vi "热敏电阻多通道数据采集 - 副本.vi"() -> ()   [LabVIEW 2015]
uses:
  <vilib>/Utility/miscctls.llb/LVRowAndColumnTypeDef.ctl
  <vilib>/addons/_office/_exclsub.llb/font.ctl
  <vilib>/addons/_office/excel.llb/Excel Easy Table (str).vi
  <vilib>/Utility/NIReport.llb/NI_report.lvclass
  Keithley 27XX/Keithley 27XX.lvlib
  <vilib>/addons/_office/NI_ReportGenerationToolkit.lvlib
panel:
  out "数据显示 3":string[][](table)
  in  "Quit":bool
  out "队列输出":refnum<queue>
  out "采集使能":bool
  out "数据显示":string[][](table)
  in  "tab":enum32{"总线检查", "配置", "数据显示"}(tab)
  in  "Keithley2750":refnum<visa-resource-name>="COM3"
  in  "总线检查":bool
  in  "温度设置":bool
  in  "编号设置":bool
  in  "清空表格":bool
  in  "暂停":bool
  in  "采集温度":bool
  in  "目标温度":string(combo)
  in  "实测温度":string
  in  "生成报告":bool
  out "通道号":i32
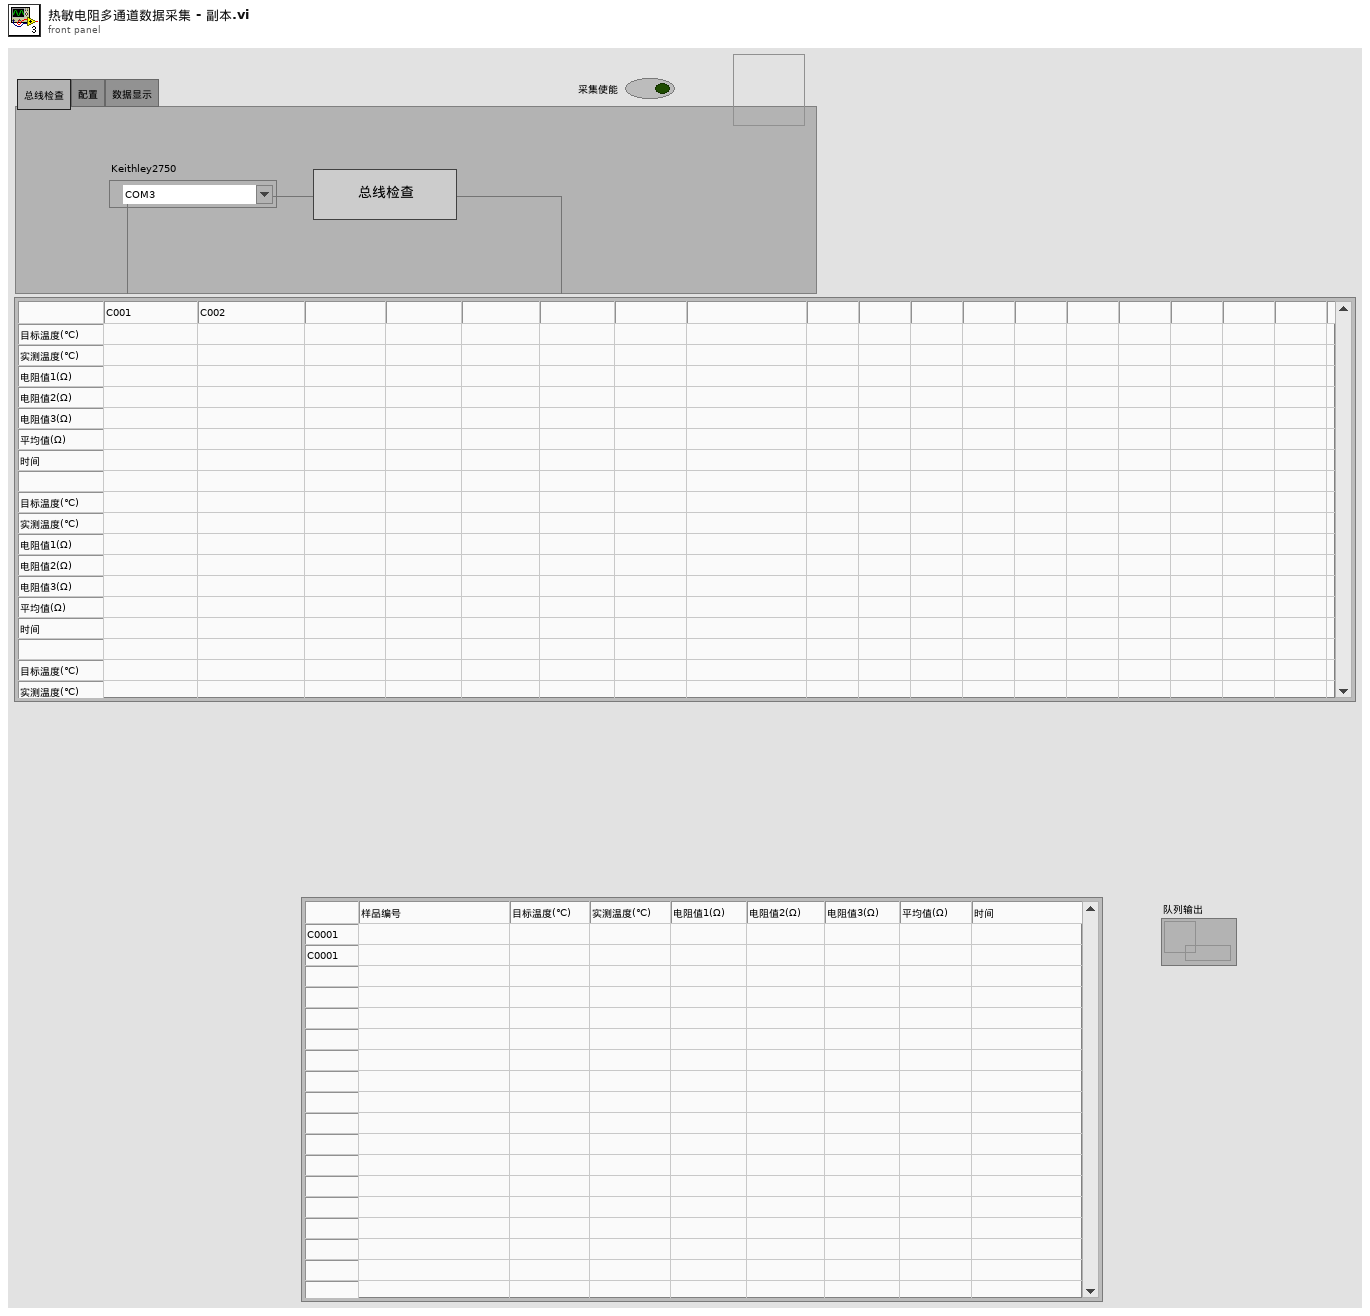
[diagram p1: front panel]
types:
  T1 = cluster{"Baud Rate (9600)":u32, "Flow Control (1: XON/XOFF)":u16, "Termination Char (0:CR)":u16}
  T2 = typedef "LVRowAndColumnTypeDef.ctl" = cluster{"Row":i32, "Column":i32}
  T3 = enum8{"Enabled", "Disabled", "Disabled and Grayed Out"}
  T4 = enum16{"maximized", "minimized", "normal", "no change"}
  T5 = enum16{"Standard Report", "HTML", "Word", "Excel"}
  T6 = typedef "NI_ReportGenerationToolkit.lvlib/font.ctl" = cluster{"font name":string, "font size":dbl, "bold":u16, "italic":u16, "underline":u16, "strike through":u16, "font color":u32}
  T7 = typedef "LVPoint32TypeDef.ctl" = cluster{"Horizontal":i32, "Vertical":i32}
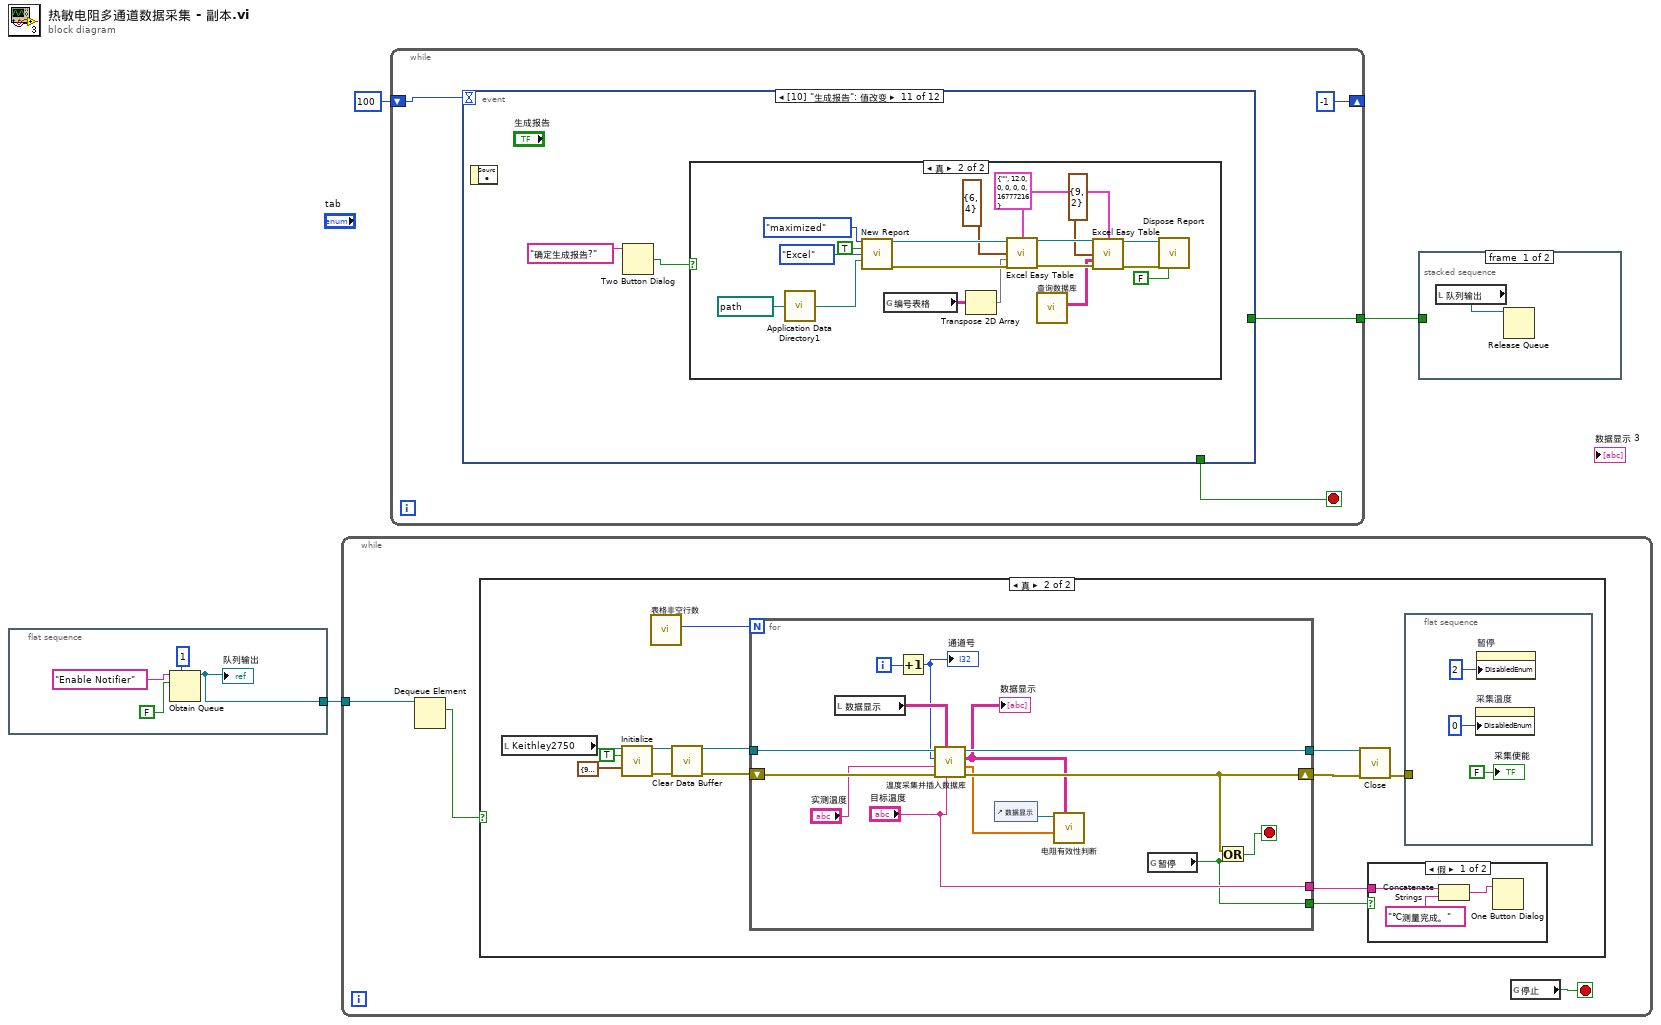
[diagram p0: block diagram]
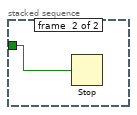
[diagram p2: hidden frame]
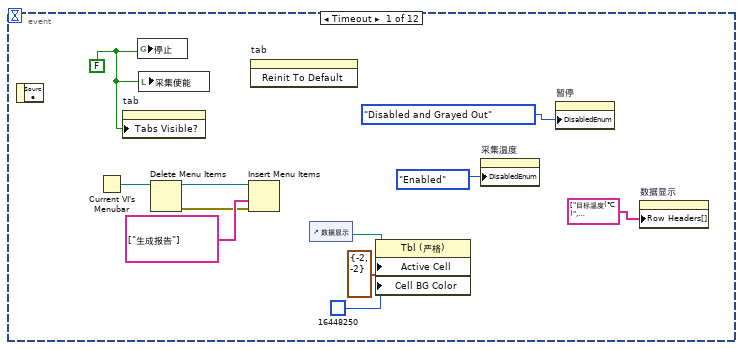
[diagram p5: hidden frame]
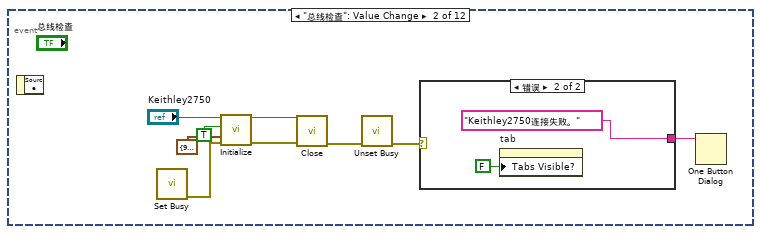
[diagram p6: hidden frame]
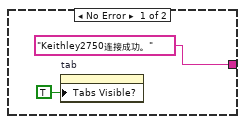
[diagram p7: hidden frame]
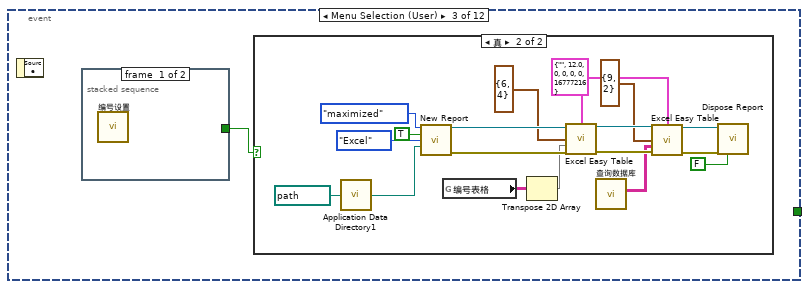
[diagram p8: hidden frame]
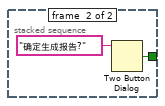
[diagram p9: hidden frame]
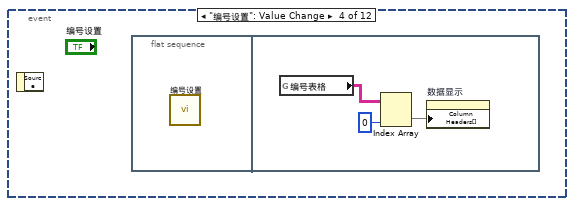
[diagram p11: hidden frame]
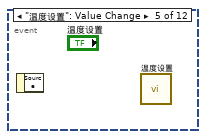
[diagram p12: hidden frame]
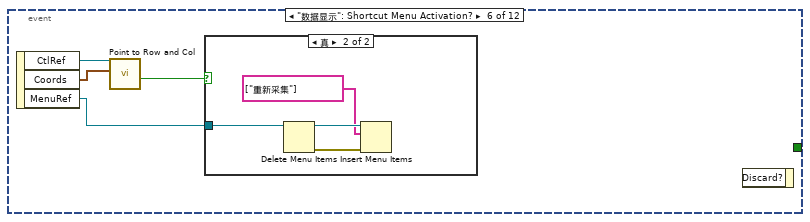
[diagram p13: hidden frame]
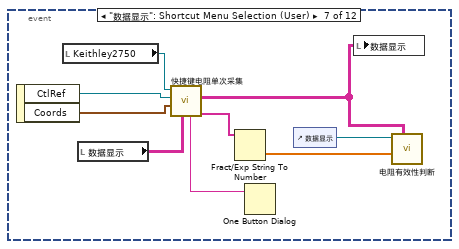
[diagram p15: hidden frame]
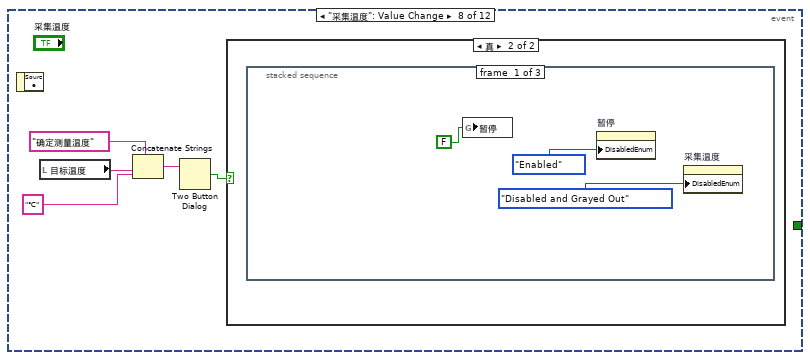
[diagram p16: hidden frame]
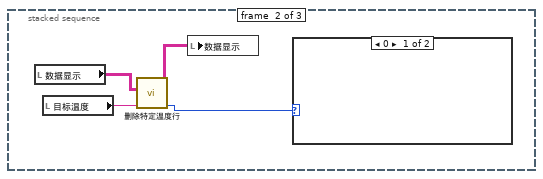
[diagram p18: hidden frame]
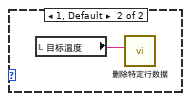
[diagram p19: hidden frame]
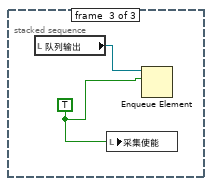
[diagram p20: hidden frame]
diagram:
  n1 = flat-sequence {
    tunnel: [w4] -> w1
    frame #0 {
      n2 = Obtain Queue(max queue size (-1, unlimited)=1 ("队列最大值（-1，无限）"), name (unnamed)="Enable Notifier", element data type=FALSE ("stop confirmed")) -> (queue out=w4:refnum<queue>)  [unwired: 2 in, 2 out]
      "队列输出" <- w4
    }
  }
  n3 = while {
    tunnel: w1 -> [w9]
    stop <- w10 stop-if-true
    n4 = Dequeue Element(queue=w9) -> (element=w8:bool)  [unwired: 2 in, 3 out]
    n5 = case shown="真" w8 {
      frame False {
      }
      frame True {
        n6 = local read "Keithley2750"() -> (w23:refnum<visa-resource-name>)
        n7 = call "Initialize.vi"("VISA resource name"=w23, "ID Query? (T: Yes)"=TRUE, "Serial Configuration"=T1 {"Baud Rate (9600)"=9600, "Flow Control (1: XON/XOFF)"=1, "Termination Char (0:CR)"=0}) -> ("VISA resource name out"=w21:refnum<visa-resource-name>, "error out"=w20:errorcluster)  [unwired: 11 in]
        n8 = call "表格非空行数.vi"() -> ("行数"=w12:i32)  [unwired: 11 in]
        n9 = call "Clear Data Buffer.vi"("VISA resource name"=w21, "error in (no error)"=w20) -> ("VISA resource name out"=w18:refnum<visa-resource-name>, "error out"=w19:errorcluster)  [unwired: 12 in]
        n10 = for {
          N: w12 -> [_]
          shift-right: [w40] -> w17
          shift-left: w19 -> [w43]
          tunnel: ["目标温度"] -> w13
          tunnel: w18 -> [w42]
          tunnel: [w41] -> w16
          tunnel: [w31] -> w11
          i -> [w32]
          stop <- w39 stop-if-true
          n11 = local read "数据显示"() -> (w34:string[][])
          n12 = Increment(x=w32) -> (x+1=w30:i32)
          "通道号" <- w30
          n13 = call "温度采集并插入数据库.vi"("目标温度"="目标温度", "数据显示1"=w34, "错误输入（无错误）"=w43, "实测温度"="实测温度", "通道号"=w30, "VISA引用句柄输入"=w42) -> ("错误输出"=w40:errorcluster, "温度值s"=w36:dbl[], "数据显示2"=w35:string[][], "VISA引用句柄输出"=w41:refnum<visa-resource-name>)  [unwired: 2 in]
          "数据显示" <- w35
          n14 = control-ref of="数据显示"() -> (w37:refnum<vi>)
          n15 = call "电阻有效性判断.vi"("数据显示"=w35, "温度值s"=w36, "Table输入"=w37) -> ()  [unwired: 9 in]
          n16 = global read "全局.vi" "暂停"() -> (w31:bool)
          n17 = Or(x=w40, y=w31) -> (x .or. y?=w39:bool)
        }
        n18 = call "Close.vi"("VISA resource name"=w16, "error in (no error)"=w17) -> ("error out"=w15:errorcluster)  [unwired: 13 in]
        n19 = case shown="假" w11 {
          tunnel: w13 -> [w26 _]
          frame False {
            n20 = Concatenate Strings(w26, "℃测量完成。") -> (w24:string)
            n21 = One Button Dialog(message=w24) -> ()  [unwired: 1 in, 1 out]
          }
          frame True {
          }
        }
        n22 = flat-sequence {
          tunnel: w15 -> [_]
          frame #0 {
            n23 = property on="采集温度" class="Bool"("DisabledEnum"=0) -> ()  [unwired: 2 in, 2 out]
            n24 = property on="暂停" class="Bool"("DisabledEnum"=2) -> ()  [unwired: 2 in, 2 out]
            "采集使能" <- FALSE ("采集使能")
          }
        }
      }
    }
    n25 = global read "全局.vi" "停止"() -> (w10:bool)
  }
  n26 = while {
    shift-right: [-1] -> _
    shift-left: 100 -> [w46]
    tunnel: [w44] -> w2
    stop <- w45 stop-if-true
    n27 = event shown="[10] \"生成报告\": 值改变" {
      selector: _ -> [_ _ _ _ _ _ _ _ _ _ _ _]
      dyn-events: _ -> [_ _ _ _ _ _ _ _ _ _ _ _]
      timeout: w46 -> [_ _ _ _ _ _ _ _ _ _ _ _]
      tunnel: [_ _ _ _ _ _ _ _ _ _ _ w154] -> w45
      tunnel: [_ _ _ _ _ _ _ _ _ _ _ w154] -> w44
      event Timeout {
        w54 = FALSE ("Excel已打开")
        n28 = event-data() -> ()  [unwired: 1 in, 1 out]
        n29 = Current VI's Menubar() -> (w56:refnum<k9>)
        n30 = property on="tab" class="TabCtl (严格)"("Tabs Visible?"=w54) -> ()  [unwired: 2 in, 2 out]
        n31 = global write "全局.vi" "停止"(w54) -> ()
        n32 = local write "采集使能"(w54) -> ()
        n33 = Delete Menu Items(9:w56) -> (0:w55:errorcluster, 3:w57:refnum<k9>)  [unwired: 3 in]
        n34 = Insert Menu Items(6:w55, 7:string[] ["生成报告"] ("L10n_item tags 1"), 9:w57) -> ()  [unwired: 3 in, 3 out]
        n35 = invoke on="tab" class="TabCtl (严格)" method="Reinit To Default"() -> ()  [unwired: 3 in, 3 out]
        n36 = control-ref of="数据显示"() -> (w51:refnum<vi>)
        n37 = property class="Tbl (严格)"(reference=w51, "Active Cell"=T2 {"Row"=-2, "Column"=-2} ("活动单元格:活动单元格"), "Cell BG Color"=u32 16448250 ("Origin BK Color")) -> ()  [unwired: 1 in, 2 out]
        n38 = property on="采集温度" class="Bool"("DisabledEnum"=T3."Enabled" ("禁用")) -> ()  [unwired: 2 in, 2 out]
        n39 = property on="暂停" class="Bool"("DisabledEnum"=T3."Disabled and Grayed Out" ("禁用")) -> ()  [unwired: 2 in, 2 out]
        n40 = property on="数据显示" class="Tbl (严格)"("Row Headers[]"=string[] ["目标温度(℃)", "实测温度(℃)", "电阻值1(Ω)", "电阻值2(Ω)", "电阻值3(Ω)", "平均值(Ω)", "时间", "", "目标温度(℃)", "实测温度(℃)", "电阻值1(Ω)", "电阻值2(Ω)", "电阻值3(Ω)", "平均值(Ω)", "时间", "", "目标温度(℃)", "实测温度(℃)", "电阻值1(Ω)", "电阻值2(Ω)", "电阻值3(Ω)", "平均值(Ω)", "时间", "", "目标温度(℃)", "实测温度(℃)", "电阻值1(Ω)", "电阻值2(Ω)", "电阻值3(Ω)", "平均值(Ω)", "时间", "", "目标温度(℃)", "实测温度(℃)", "电阻值1(Ω)", "电阻值2(Ω)", "电阻值3(Ω)", "平均值(Ω)", "时间", "", "目标温度(℃)", "实测温度(℃)", "电阻值1(Ω)", "电阻值2(Ω)", "电阻值3(Ω)", "平均值(Ω)", "时间", "", "目标温度(℃)", "实测温度(℃)", "电阻值1(Ω)", "电阻值2(Ω)", "电阻值3(Ω)", "平均值(Ω)", "时间", "", "目标温度(℃)", "实测温度(℃)", "电阻值1(Ω)", "电阻值2(Ω)", "电阻值3(Ω)", "平均值(Ω)", "时间", "", "目标温度(℃)", "实测温度(℃)", "电阻值1(Ω)", "电阻值2(Ω)", "电阻值3(Ω)", "平均值(Ω)", "时间", "", "目标温度(℃)", "实测温度(℃)", "电阻值1(Ω)", "电阻值2(Ω)", "电阻值3(Ω)", "平均值(Ω)", "时间", "", "目标温度(℃)", "实测温度(℃)", "电阻值1(Ω)", "电阻值2(Ω)", "电阻值3(Ω)", "平均值(Ω)", "时间", "", "目标温度(℃)", "实测温度(℃)", "电阻值1(Ω)", "电阻值2(Ω)", "电阻值3(Ω)", "平均值(Ω)", "时间", "", "目标温度(℃)", "实测温度(℃)", "电阻值1(Ω)", "电阻值2(Ω)", "电阻值3(Ω)", "平均值(Ω)", "时间", "", "目标温度(℃)", "实测温度(℃)", "电阻值1(Ω)", "电阻值2(Ω)", "电阻值3(Ω)", "平均值(Ω)", "时间", "", "目标温度(℃)", "实测温度(℃)", "电阻值1(Ω)", "电阻值2(Ω)", "电阻值3(Ω)", "平均值(Ω)", "时间", "", "目标温度(℃)", "实测温度(℃)", "电阻值1(Ω)", "电阻值2(Ω)", "电阻值3(Ω)", "平均值(Ω)", "时间", "", "目标温度(℃)", "实测温度(℃)", "电阻值1(Ω)", "电阻值2(Ω)", "电阻值3(Ω)", "平均值(Ω)", "时间", "", "目标温度(℃)", "实测温度(℃)", "电阻值1(Ω)", "电阻值2(Ω)", "电阻值3(Ω)", "平均值(Ω)", "时间", "", "目标温度(℃)", "实测温度(℃)", "电阻值1(Ω)", "电阻值2(Ω)", "电阻值3(Ω)", "平均值(Ω)", "时间", "", "目标温度(℃)", "实测温度(℃)", "电阻值1(Ω)", "电阻值2(Ω)", "电阻值3(Ω)", "平均值(Ω)", "时间", "", "目标温度(℃)", "实测温度(℃)", "电阻值1(Ω)", "电阻值2(Ω)", "电阻值3(Ω)", "平均值(Ω)", "时间", "", "目标温度(℃)", "实测温度(℃)", "电阻值1(Ω)", "电阻值2(Ω)", "电阻值3(Ω)", "平均值(Ω)", "时间", "", "目标温度(℃)", "实测温度(℃)", "电阻值1(Ω)", "电阻值2(Ω)", "电阻值3(Ω)", "平均值(Ω)", "时间", "", "目标温度(℃)", "实测温度(℃)", "电阻值1(Ω)", "电阻值2(Ω)", "电阻值3(Ω)", "平均值(Ω)", "时间", "", "目标温度(℃)", "实测温度(℃)", "电阻值1(Ω)", "电阻值2(Ω)", "电阻值3(Ω)", "平均值(Ω)", "时间", "", "目标温度(℃)", "实测温度(℃)", "电阻值1(Ω)", "电阻值2(Ω)", "电阻值3(Ω)", "平均值(Ω)", "时间", "", "目标温度(℃)", "实测温度(℃)", "电阻值1(Ω)", "电阻值2(Ω)", "电阻值3(Ω)", "平均值(Ω)", "时间", "", "目标温度(℃)", "实测温度(℃)", "电阻值1(Ω)", "电阻值2(Ω)", "电阻值3(Ω)", "平均值(Ω)", "时间", "", "目标温度(℃)", "实测温度(℃)", "电阻值1(Ω)", "电阻值2(Ω)", "电阻值3(Ω)", "平均值(Ω)", "时间", "", "目标温度(℃)", "实测温度(℃)", "电阻值1(Ω)", "电阻值2(Ω)", "电阻值3(Ω)", "平均值(Ω)", "时间", "", "目标温度(℃)", "实测温度(℃)", "电阻值1(Ω)", "电阻值2(Ω)", "电阻值3(Ω)", "平均值(Ω)", "时间", "", "目标温度(℃)", "实测温度(℃)", "电阻值1(Ω)", "电阻值2(Ω)", "电阻值3(Ω)", "平均值(Ω)", "时间", "", "目标温度(℃)", "实测温度(℃)", "电阻值1(Ω)", "电阻值2(Ω)", "电阻值3(Ω)", "平均值(Ω)", "时间", "", "目标温度(℃)", "实测温度(℃)", "电阻值1(Ω)", "电阻值2(Ω)", "电阻值3(Ω)", "平均值(Ω)", "时间", "", "目标温度(℃)", "实测温度(℃)", "电阻值1(Ω)", "电阻值2(Ω)", "电阻值3(Ω)", "平均值(Ω)", "时间", "", "目标温度(℃)", "实测温度(℃)", "电阻值1(Ω)", "电阻值2(Ω)", "电阻值3(Ω)", "平均值(Ω)", "时间", "", "目标温度(℃)", "实测温度(℃)", "电阻值1(Ω)", "电阻值2(Ω)", "电阻值3(Ω)", "平均值(Ω)", "时间", "", "目标温度(℃)", "实测温度(℃)", "电阻值1(Ω)", "电阻值2(Ω)", "电阻值3(Ω)", "平均值(Ω)", "时间", "", "目标温度(℃)", "实测温度(℃)", "电阻值1(Ω)", "电阻值2(Ω)", "电阻值3(Ω)", "平均值(Ω)", "时间", "", "目标温度(℃)", "实测温度(℃)", "电阻值1(Ω)", "电阻值2(Ω)", "电阻值3(Ω)", "平均值(Ω)", "时间", "", "目标温度(℃)", "实测温度(℃)", "电阻值1(Ω)", "电阻值2(Ω)", "电阻值3(Ω)", "平均值(Ω)", "时间", ""] ("数组")) -> ()  [unwired: 2 in, 2 out]
      }
      event "总线检查": Value Change {
        n41 = event-data() -> ()  [unwired: 1 in, 1 out]
        n42 = call <vilib>:"Set Busy.vi"() -> ("error out"=w63:errorcluster)  [unwired: 10 in, 1 out]
        n43 = call "Initialize.vi"("VISA resource name"="Keithley2750", "ID Query? (T: Yes)"=TRUE, "Serial Configuration"=T1 {"Baud Rate (9600)"=9600, "Flow Control (1: XON/XOFF)"=1, "Termination Char (0:CR)"=0}, "error in (no error)"=w63) -> ("VISA resource name out"=w65:refnum<visa-resource-name>, "error out"=w64:errorcluster)  [unwired: 10 in]
        n44 = call "Close.vi"("VISA resource name"=w65, "error in (no error)"=w64) -> ("error out"=w62:errorcluster)  [unwired: 13 in]
        n45 = call <vilib>:"Unset Busy.vi"("error in (no error)"=w62) -> ("error out"=w61:errorcluster)  [unwired: 10 in]
        n46 = case shown="错误" w61 {
          tunnel: ["Keithley2750连接成功。" ("消息") "Keithley2750连接失败。" ("消息")] -> w60
          frame No Error {
            n47 = property on="tab" class="TabCtl (严格)"("Tabs Visible?"=TRUE ("选项卡可见？")) -> ()  [unwired: 2 in, 2 out]
          }
          frame Error {
            n48 = property on="tab" class="TabCtl (严格)"("Tabs Visible?"=FALSE ("选项卡可见？")) -> ()  [unwired: 2 in, 2 out]
          }
        }
        n49 = One Button Dialog(message=w60) -> ()  [unwired: 1 in, 1 out]
      }
      event Menu Selection (User) {
        n50 = event-data() -> ()  [unwired: 1 in, 1 out]
        n51 = stacked-sequence {
          tunnel: [_ w73] -> w72
          frame #0 {
            n52 = call "编号设置.vi"() -> ()  [unwired: 12 in]
          }
          frame #1 {
            n53 = Two Button Dialog(message="确定生成报告?" ("消息")) -> (T button?=w73:bool)  [unwired: 2 in]
          }
        }
        n54 = case shown="真" w72 {
          frame False {
          }
          frame True {
            w77 = T6 {"font name"="", "font size"=12.0, "bold"=0, "italic"=0, "underline"=0, "strike through"=0, "font color"=16777216} ("font")
            n55 = call "Application Data Directory1.vi"("Relative path (.)"=path "模板.xls") -> ("Application Directory (+ Relative)"=w75:path)
            n56 = call <vilib>:"New Report.vi"("window state (normal)"=T4."maximized", "display alerts? (F)"=TRUE, "report type"=T5."Excel", "template (empty)"=w75) -> ("report out"=w87:refnum<class "NI_report.lvclass">, "error out"=w88:errorcluster)  [unwired: 10 in]
            n57 = global read "全局.vi" "编号表格"() -> (w86:string[][])
            n58 = Transpose 2D Array(2D array=w86) -> (transposed array=w84:string[][])
            n59 = call-poly <vilib>:"Excel Easy Table.vi"("report in"=w87, "font"=w77, "start (0, 0)"=cluster{"row":i32, "column":i32} {"row"=6, "column"=4}, "text data"=w84, "error in (no error)"=w88) -> ("report out"=w83:refnum<class "NI_report.lvclass">, "error out"=w82:errorcluster)  [unwired: 6 in, 3 out]
            n60 = call "查询数据库.vi"() -> ("数据"=w78:string[][])  [unwired: 11 in]
            n61 = call-poly <vilib>:"Excel Easy Table.vi"("report in"=w83, "font"=w77, "start (0, 0)"=cluster{"row":i32, "column":i32} {"row"=9, "column"=2}, "text data"=w78, "error in (no error)"=w82) -> ("report out"=w81:refnum<class "NI_report.lvclass">, "error out"=w80:errorcluster)  [unwired: 6 in, 3 out]
            n62 = call-dynamic "Dispose Report.vi"("report in"=w81, "error in (no error)"=w80, "close report? (T)"=FALSE) -> ()  [unwired: 12 in, 1 out]
          }
        }
      }
      event "编号设置": Value Change {
        n63 = event-data() -> ()  [unwired: 1 in, 1 out]
        n64 = flat-sequence {
          frame #0 {
            n65 = call "编号设置.vi"() -> ()  [unwired: 12 in]
          }
          frame #1 {
            n66 = global read "全局.vi" "编号表格"() -> (w93:string[][])
            n67 = Index Array(array=w93, index (col)=0 ("禁用的索引 (列)")) -> (element=w95:string[])  [unwired: 1 in]
            n68 = property on="数据显示" class="Tbl (严格)"("Column Headers[]"=w95) -> ()  [unwired: 2 in, 2 out]
          }
        }
      }
      event "温度设置": Value Change {
        n69 = event-data() -> ()  [unwired: 1 in, 1 out]
        n70 = call "温度设置.vi"() -> ()  [unwired: 12 in]
      }
      event "数据显示": Shortcut Menu Activation? {
        n71 = event-data() -> ("CtlRef"=w98:refnum<vi>, "Coords"=w99:T7, "MenuRef"=w96:refnum<k9>)  [unwired: 1 in]
        n72 = call "Point to Row and Col.vi"("点"=w99, "Table Ref In"=w98) -> ("边界内？"=w97:bool)  [unwired: 6 in, 3 out]
        n73 = case shown="真" w97 {
          tunnel: w96 -> [_ w101]
          frame False {
          }
          frame True {
            n74 = Delete Menu Items(9:w101) -> (0:w103:errorcluster, 3:w102:refnum<k9>)  [unwired: 3 in]
            n75 = Insert Menu Items(6:w103, 8:string[] ["重新采集"] ("项名称"), 9:w102) -> ()  [unwired: 3 in, 3 out]
          }
        }
        n76 = event-data() -> ()  [unwired: 2 in, 1 out]
      }
      event "数据显示": Shortcut Menu Selection (User) {
        n77 = event-data() -> ("CtlRef"=w111:refnum<vi>, "Coords"=w110:T7)  [unwired: 1 in]
        n78 = local read "Keithley2750"() -> (w112:refnum<visa-resource-name>)
        n79 = local read "数据显示"() -> (w109:string[][])
        n80 = call "快捷键电阻单次采集.vi"("数据显示1"=w109, "Coords"=w110, "CtlRef"=w111, "Keithley2705"=w112) -> ("采集值+平均值"=w108:string[], "数据显示2"=w106:string[][], "完成对话框"=w104:string)  [unwired: 5 in]
        n81 = Fract/Exp String To Number(string=w108) -> (number=w107:dbl[])  [unwired: 3 in, 1 out]
        n82 = One Button Dialog(message=w104) -> ()  [unwired: 1 in, 1 out]
        n83 = control-ref of="数据显示"() -> (w105:refnum<vi>)
        n84 = local write "数据显示"(w106) -> ()
        n85 = call "电阻有效性判断.vi"("数据显示"=w106, "温度值s"=w107, "Table输入"=w105) -> ()  [unwired: 9 in]
      }
      event "采集温度": Value Change {
        n86 = event-data() -> ()  [unwired: 1 in, 1 out]
        n87 = local read "目标温度"() -> (w115:string)
        n88 = Concatenate Strings("确定测量温度", w115, "℃") -> (w117:string)
        n89 = Two Button Dialog(message=w117) -> (T button?=w113:bool)  [unwired: 2 in]
        n90 = case shown="真" w113 {
          frame False {
          }
          frame True {
            n91 = stacked-sequence {
              frame #0 {
                n92 = global write "全局.vi" "暂停"(FALSE ("暂停")) -> ()
                n93 = property on="暂停" class="Bool"("DisabledEnum"=T3."Enabled" ("禁用")) -> ()  [unwired: 2 in, 2 out]
                n94 = property on="采集温度" class="Bool"("DisabledEnum"=T3."Disabled and Grayed Out" ("禁用")) -> ()  [unwired: 2 in, 2 out]
              }
              frame #1 {
                n95 = local read "数据显示"() -> (w124:string[][])
                n96 = local read "目标温度"() -> (w122:string)
                n97 = call "删除特定温度行.vi"("匹配元素"=w122, "数据显示1"=w124) -> ("匹配数量"=w121:i32, "数据显示2"=w123:string[][])  [unwired: 7 in, 1 out]
                n98 = local write "数据显示"(w123) -> ()
                n99 = case shown="0" w121 {
                  frame 0 {
                  }
                  frame 1, Default {
                    n100 = local read "目标温度"() -> (w125:string)
                    n101 = call "删除特定行数据.vi"("目标温度"=w125) -> ()  [unwired: 11 in]
                  }
                }
              }
              frame #2 {
                w126 = TRUE ("采集使能")
                n102 = local read "队列输出"() -> (w127:refnum<queue>)
                n103 = local write "采集使能"(w126) -> ()
                n104 = Enqueue Element(queue=w127, element=w126) -> ()  [unwired: 2 in, 3 out]
              }
            }
          }
        }
      }
      event "暂停": Value Change {
        n105 = event-data() -> ()  [unwired: 1 in, 1 out]
        n106 = flat-sequence {
          frame #0 {
            n107 = global write "全局.vi" "暂停"(TRUE ("暂停")) -> ()
          }
          frame #1 {
            w131 = FALSE ("采集使能")
            n108 = local read "队列输出"() -> (w132:refnum<queue>)
            n109 = local write "采集使能"(w131) -> ()
            n110 = Enqueue Element(queue=w132, element=w131) -> ()  [unwired: 2 in, 3 out]
          }
        }
        n111 = property on="暂停" class="Bool"("DisabledEnum"=T3."Disabled and Grayed Out" ("禁用")) -> ()  [unwired: 2 in, 2 out]
        n112 = property on="采集温度" class="Bool"("DisabledEnum"=T3."Enabled" ("禁用")) -> ()  [unwired: 2 in, 2 out]
      }
      event "清空表格": Value Change {
        n113 = event-data() -> ()  [unwired: 1 in, 1 out]
        n114 = local write "数据显示"(string[][] [] ("数据显示")) -> ()
      }
      event "生成报告": Value Change {
        n115 = event-data() -> ()  [unwired: 1 in, 1 out]
        n116 = Two Button Dialog(message="确定生成报告?" ("消息")) -> (T button?=w134:bool)  [unwired: 2 in]
        n117 = case shown="真" w134 {
          frame False {
          }
          frame True {
            w138 = T6 {"font name"="", "font size"=12.0, "bold"=0, "italic"=0, "underline"=0, "strike through"=0, "font color"=16777216} ("font")
            n118 = call "Application Data Directory1.vi"("Relative path (.)"=path "模板.xls") -> ("Application Directory (+ Relative)"=w136:path)
            n119 = call <vilib>:"New Report.vi"("window state (normal)"=T4."maximized", "display alerts? (F)"=TRUE, "report type"=T5."Excel", "template (empty)"=w136) -> ("report out"=w148:refnum<class "NI_report.lvclass">, "error out"=w149:errorcluster)  [unwired: 10 in]
            n120 = global read "全局.vi" "编号表格"() -> (w147:string[][])
            n121 = Transpose 2D Array(2D array=w147) -> (transposed array=w145:string[][])
            n122 = call-poly <vilib>:"Excel Easy Table.vi"("report in"=w148, "font"=w138, "start (0, 0)"=cluster{"row":i32, "column":i32} {"row"=6, "column"=4}, "text data"=w145, "error in (no error)"=w149) -> ("report out"=w144:refnum<class "NI_report.lvclass">, "error out"=w143:errorcluster)  [unwired: 6 in, 3 out]
            n123 = call "查询数据库.vi"() -> ("数据"=w139:string[][])  [unwired: 11 in]
            n124 = call-poly <vilib>:"Excel Easy Table.vi"("report in"=w144, "font"=w138, "start (0, 0)"=cluster{"row":i32, "column":i32} {"row"=9, "column"=2}, "text data"=w139, "error in (no error)"=w143) -> ("report out"=w142:refnum<class "NI_report.lvclass">, "error out"=w141:errorcluster)  [unwired: 6 in, 3 out]
            n125 = call-dynamic "Dispose Report.vi"("report in"=w142, "error in (no error)"=w141, "close report? (T)"=FALSE) -> ()  [unwired: 12 in, 1 out]
          }
        }
      }
      event "Quit": Value Change {
        w154 = TRUE
        n126 = event-data() -> ()  [unwired: 1 in, 1 out]
        n127 = global write "全局.vi" "停止"(w154) -> ()
      }
    }
  }
  n128 = stacked-sequence {
    tunnel: w2 -> [_ w156]
    frame #0 {
      n129 = local read "队列输出"() -> (w155:refnum<queue>)
      n130 = Release Queue(queue=w155) -> ()  [unwired: 2 in, 3 out]
    }
    frame #1 {
      n131 = Stop(stop? (T)=w156) -> ()
    }
  }
